vi "Server_Save.vi"(8 "error in (no error)":errorcluster, 9 "Code":string, 10 "Name":string="file.py", 11 "Server":path) -> (0 "error out":errorcluster)   [LabVIEW 2020]
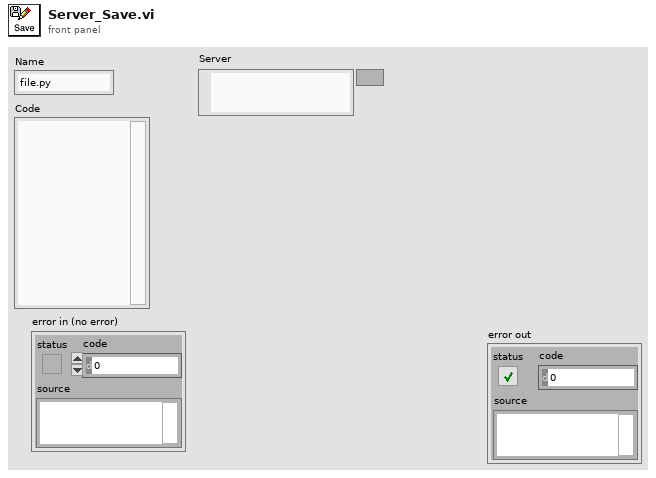
[diagram p1: front panel]
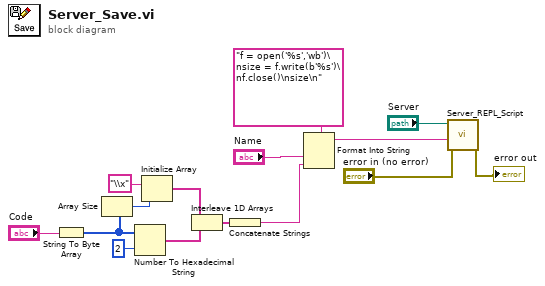
[diagram p0: block diagram]
diagram:
  n1 = String To Byte Array(string="Code") -> (unsigned byte array=w13:u8[])
  n2 = Array Size(array=w13) -> (size(s)=w12:i32)
  n3 = Number To Hexadecimal String(1:i16 2 ("width (-)"), 2:w13) -> (0:w10:string[])
  n4 = Initialize Array("\\x", w12) -> (w11:string[])
  n5 = Interleave 1D Arrays(w11, w10) -> (w9:string[])
  n6 = Concatenate Strings(w9) -> (w8:string)
  n7 = Format Into String(format string="f = open('%s','wb')\nsize = f.write(b'%s')\nf.close()\nsize\n", "Name", w8) -> (resulting string=w1:string)  [unwired: 2 in, 1 out]
  n8 = call "Server_REPL_Script.vi"("error in (no error)"="error in (no error)", "Code"=w1, "Server"="Server") -> ("error out"=→"error out":errorcluster)  [unwired: 8 in]
